vi "Add Input Type to JSON.vi"(8 "error in (no error)":errorcluster, 10 "input cfg JSON":string, 11 "input type":T1 caption="master clock source") -> (0 "error out":errorcluster, 3 "input cfg JSON":string)   [LabVIEW 2022 SP3, in "input cfg file.lvlib"]
uses:
  input cfg file.lvlib
  controls/input type.ctl
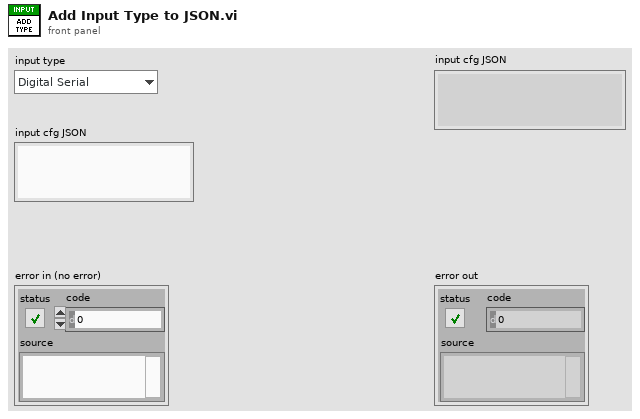
[diagram p1: front panel]
types:
  T1 = typedef "input type.ctl" = enum32{"Digital Serial", "PDM"}
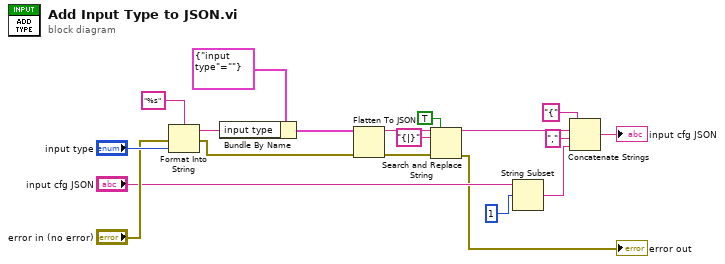
[diagram p0: block diagram]
diagram:
  n1 = Format Into String(format string="%s", error in="error in (no error)", "input type") -> (resulting string=w16:string, error out=w10:errorcluster)  [unwired: 1 in]
  n2 = Bundle By Name(cluster=cluster{"input type":string} {"input type"=""}, "input type"=w16) -> (w15:cluster{"input type":string})
  n3 = Flatten To JSON(anything=w15, error in (no error)=w10) -> (JSON string=w14:string, 11:w9:errorcluster)  [unwired: 1 in]
  n4 = Search and Replace String(replace all?=TRUE ("replace all? (F)"), input string=w14, search string="{|}", error in=w9) -> (result string=w4:string, error out=→"error out":errorcluster)  [unwired: 4 in, 2 out]
  n5 = String Subset(string="input cfg JSON", offset (0)=1) -> (substring=w5:string)  [unwired: 1 in]
  n6 = Concatenate Strings("{" ("string"), w4, "," ("string"), w5) -> (→"input cfg JSON":string)
